vi "HFRR ADV v08 new software.vi"() -> ()   [LabVIEW 2025] (continued)
                  n3105 = Concatenate Strings(w4140, "=" ("string")) -> (→"String 37":string)
                }
                frame 43 {
                  n3106 = property on="HCF 2" class="DigNum (strict)"("Caption.Text"=w4143) -> ()  [unwired: 2 in, 2 out]
                  n3107 = property on="HCF" class="DigNum (strict)"("Caption.Text"=w4143) -> ()  [unwired: 2 in, 2 out]
                  n3108 = Concatenate Strings(w4143, "=" ("string")) -> (→"String 38":string)
                }
                frame 44 {
                  n3109 = Concatenate Strings(w4145, "=" ("string")) -> (→"String 39":string)
                  n3110 = property on="WS1.4 2" class="DigNum (strict)"("Caption.Text"=w4145) -> ()  [unwired: 2 in, 2 out]
                  n3111 = property on="WS1.4" class="DigNum (strict)"("Caption.Text"=w4145) -> ()  [unwired: 2 in, 2 out]
                }
                frame 45 {
                  n3112 = property on="Save Results" class="Bool (strict)"("Boolean Text.Text"=w4147) -> ()  [unwired: 2 in, 2 out]
                }
                frame 46 {
                  n3113 = local write "S 47"(w4148) -> ()
                }
                frame 47 {
                  n3114 = local write "S 48"(w4149) -> ()
                }
                frame 48 {
                  n3115 = local write "S 49"(w4150) -> ()
                }
                frame 49 {
                  n3116 = local write "S 50"(w4151) -> ()
                }
                frame 50 {
                  n3117 = local write "S 51"(w4152) -> ()
                }
                frame 51 {
                  n3118 = local write "S 52"(w4153) -> ()
                }
                frame 52 {
                  n3119 = local write "S 53"(w4154) -> ()
                }
                frame 53 {
                  n3120 = local write "S 54"(w4155) -> ()
                }
                frame 54 {
                  n3121 = local write "S 55"(w4156) -> ()
                }
                frame 55 {
                  n3122 = local write "S 56"(w4157) -> ()
                }
                frame 56 {
                  n3123 = local write "S 57"(w4158) -> ()
                }
                frame 57 {
                  n3124 = local write "S 58"(w4159) -> ()
                }
                frame 58 {
                  n3125 = local write "S 59"(w4160) -> ()
                }
                frame 59 {
                  n3126 = local write "S 60"(w4161) -> ()
                }
                frame 60 {
                  n3127 = local write "S 62"(w4162) -> ()
                }
                frame 61 {
                  n3128 = local write "S 63"(w4163) -> ()
                }
                frame 62 {
                  n3129 = local write "S 64"(w4164) -> ()
                }
                frame 63 {
                  n3130 = local write "S 65"(w4165) -> ()
                }
                frame 64 {
                  n3131 = local write "S 66"(w4166) -> ()
                }
                frame 65 {
                  n3132 = local write "S 67"(w4167) -> ()
                }
                frame 66 {
                  n3133 = local write "S 68"(w4168) -> ()
                }
                frame 67 {
                  n3134 = local write "S 69"(w4169) -> ()
                }
                frame 68 {
                  n3135 = local write "S 70"(w4170) -> ()
                }
                frame 69 {
                  n3136 = local write "S 71"(w4171) -> ()
                }
                frame 70 {
                  n3137 = local write "S 72"(w4172) -> ()
                }
                frame 71 {
                  n3138 = local write "S 73"(w4173) -> ()
                }
                frame 72 {
                  n3139 = local write "S 74"(w4174) -> ()
                }
                frame 73 {
                  n3140 = local write "S 75"(w4175) -> ()
                }
                frame 74 {
                  n3141 = local write "S 76"(w4176) -> ()
                }
                frame 75 {
                  n3142 = local write "S 77"(w4177) -> ()
                }
                frame 76 {
                  n3143 = local write "S 78"(w4178) -> ()
                }
                frame 77 {
                  n3144 = local write "S 79"(w4179) -> ()
                }
                frame 79 {
                  n3145 = property on="Sample Temperature ( °C )" class="XYGraph (strict)"("Y Scale.Name Label.Text"=w4180) -> ()  [unwired: 2 in, 2 out]
                }
                frame 80 {
                  n3146 = local write "S 81"(w4181) -> ()
                  n3147 = property on="Humidity ( %RH )" class="XYGraph (strict)"("Y Scale.Name Label.Text"=w4181) -> ()  [unwired: 2 in, 2 out]
                }
                frame 78 {
                  n3148 = property on="Air Temperature  ( °C )" class="XYGraph (strict)"("X Scale.Name Label.Text"=w4182) -> ()  [unwired: 2 in, 2 out]
                  n3149 = property on="Humidity ( %RH )" class="XYGraph (strict)"("X Scale.Name Label.Text"=w4182) -> ()  [unwired: 2 in, 2 out]
                  n3150 = property on="Sample Temperature ( °C )" class="XYGraph (strict)"("X Scale.Name Label.Text"=w4182) -> ()  [unwired: 2 in, 2 out]
                  n3151 = property on="Coefficient Of Friction" class="XYGraph (strict)"("X Scale.Name Label.Text"=w4182) -> ()  [unwired: 2 in, 2 out]
                }
                frame 81 {
                  n3152 = property on="Air Temperature  ( °C )" class="XYGraph (strict)"("Y Scale.Name Label.Text"=w4183) -> ()  [unwired: 2 in, 2 out]
                }
                frame 82 {
                  n3153 = local write "S 84"(w4184) -> ()
                }
                frame 83 {
                  n3154 = local write "S 85"(w4185) -> ()
                }
                frame 84 {
                  n3155 = local write "S 86"(w4186) -> ()
                }
                frame 85 {
                  n3156 = local write "S 87"(w4187) -> ()
                }
                frame 86 {
                  n3157 = local write "S 88"(w4188) -> ()
                }
                frame 87 {
                }
                frame 88 {
                  n3158 = local write "S 90"(w4190) -> ()
                }
                frame 89 {
                  n3159 = local write "S 91"(w4191) -> ()
                }
                frame 90 {
                  n3160 = local write "S 92"(w4192) -> ()
                }
                frame 91 {
                  n3161 = local write "S 93"(w4193) -> ()
                }
                frame 92 {
                  n3162 = local write "S 94"(w4194) -> ()
                }
                frame 93 {
                  n3163 = local write "S 95"(w4195) -> ()
                }
                frame 94 {
                  n3164 = local write "S 96"(w4196) -> ()
                }
                frame 95 {
                  n3165 = local write "S 97"(w4197) -> ()
                }
                frame 96 {
                  n3166 = local write "S 98"(w4198) -> ()
                }
                frame 97 {
                  n3167 = local write "S 99"(w4199) -> ()
                }
                frame 98 {
                  n3168 = local write "S 100"(w4200) -> ()
                }
                frame 99 {
                  n3169 = local write "S 101"(w4201) -> ()
                }
                frame 100 {
                  n3170 = local write "S 102"(w4202) -> ()
                }
                frame 101 {
                  n3171 = local write "S 103"(w4203) -> ()
                }
                frame 102 {
                  n3172 = local write "S 104"(w4204) -> ()
                }
                frame 103 {
                  n3173 = local write "S 105"(w4205) -> ()
                }
                frame 104 {
                  n3174 = local write "S 106"(w4206) -> ()
                }
                frame 105 {
                }
                frame 106 {
                  n3175 = property on="OK Button 17" class="Bool (strict)"("Boolean Text.Text"=w4207) -> ()  [unwired: 2 in, 2 out]
                }
                frame 107 {
                  n3176 = property on="OK Button 16" class="Bool (strict)"("Boolean Text.Text"=w4208) -> ()  [unwired: 2 in, 2 out]
                }
                frame 108 {
                  n3177 = property on="TITTLE" class="Str"("Caption.Text"=w4209) -> ()  [unwired: 2 in, 2 out]
                }
                frame 109 {
                  "String 30" <- w4210
                }
                frame 110 {
                  n3178 = property on="Test Date" class="Str"("Caption.Text"=w4211) -> ()  [unwired: 2 in, 2 out]
                  "String 31" <- w4211
                }
                frame 111 {
                  n3179 = property on="Sample ID" class="Str"("Caption.Text"=w4212) -> ()  [unwired: 2 in, 2 out]
                  "String 32" <- w4212
                }
                frame 112 {
                  n3180 = property on="Tested by" class="Str"("Caption.Text"=w4213) -> ()  [unwired: 2 in, 2 out]
                  "String 33" <- w4213
                }
                frame 113 {
                  n3181 = property on="System Configured Printers 2" class="Arr (strict)"("Caption.Text"=w4214) -> ()  [unwired: 2 in, 2 out]
                }
                frame 114 {
                  n3182 = property on="Selected Printer" class="Str"("Caption.Text"=w4215) -> ()  [unwired: 2 in, 2 out]
                }
                frame 115 {
                  n3183 = property on="Select Printer 3" class="DigNum (strict)"("Caption.Text"=w4216) -> ()  [unwired: 2 in, 2 out]
                }
                frame 116 {
                  n3184 = property on="Print" class="Bool (strict)"("Boolean Text.Text"=w4217) -> ()  [unwired: 2 in, 2 out]
                }
                frame 117 {
                  "String 41" <- w4218
                }
                frame 118 {
                  n3185 = property on="tested by" class="Str"("Caption.Text"=w4219) -> ()  [unwired: 2 in, 2 out]
                }
                frame 119 {
                }
                frame 120 {
                  n3186 = property on="Export" class="Bool (strict)"("Boolean Text.Text"=w4220) -> ()  [unwired: 2 in, 2 out]
                }
                frame 121 {
                  n3187 = property on="TEMP INTERCEPT:" class="DigNum (strict)"("Caption.Text"=w4221) -> ()  [unwired: 2 in, 2 out]
                }
                frame 122 {
                  n3188 = property on="AIR TEMP INTERCEPT:" class="DigNum (strict)"("Caption.Text"=w4222) -> ()  [unwired: 2 in, 2 out]
                }
                frame 123 {
                  n3189 = property on="Select File Type" class="Enum (strict)"("Caption.Text"=w4223) -> ()  [unwired: 2 in, 2 out]
                }
                frame 124 {
                  n3190 = property on="s.NO" class="Str"("Caption.Text"=w4224) -> ()  [unwired: 2 in, 2 out]
                  "String 45" <- w4224
                }
                frame 125 {
                  n3191 = property on="trip1 8" class="Bool (strict)"("Boolean Text.Text"=w4225) -> ()  [unwired: 2 in, 2 out]
                }
                frame 126, Default {
                }
              }
            }
          }
          frame #1 {
            w4233 = TRUE ("Visible")
            n3192 = local read "S 91"() -> (w4250:string)
            n3193 = local read "S 90"() -> (w4249:string)
            n3194 = local read "S 88"() -> (w4248:string)
            n3195 = property on="File Path" class="Path"("Caption.Text"=w4249) -> ()  [unwired: 2 in, 2 out]
            n3196 = property on="SrvM CP" class="Bool (strict)"("Boolean Text.Text"=w4248) -> ()  [unwired: 2 in, 2 out]
            n3197 = local read "S 71"() -> (w4243:string)
            n3198 = local read "S 86"() -> (w4245:string)
            n3199 = local read "S 85"() -> (w4246:string)
            n3200 = local read "S 87"() -> (w4244:string)
            n3201 = local read "S 84"() -> (w4247:string)
            n3202 = local read "S 103"() -> (w4232:string)
            n3203 = local read "S 104"() -> (w4231:string)
            n3204 = property on="ENTER THE NEW PASSWORD" class="Str"("Caption.Text"=w4244) -> ()  [unwired: 2 in, 2 out]
            n3205 = property on="Password" class="Str"("Caption.Text"=w4246) -> ()  [unwired: 2 in, 2 out]
            n3206 = property on="ENTER CURRENT PASSWORD" class="Str"("Caption.Text"=w4245) -> ()  [unwired: 2 in, 2 out]
            n3207 = property on="EDIT" class="Bool (strict)"("Boolean Text.Text"=w4243) -> ()  [unwired: 2 in, 2 out]
            n3208 = property on="SAVE" class="Bool (strict)"("Boolean Text.Text"=w4247) -> ()  [unwired: 2 in, 2 out]
            n3209 = Build Array(w4232, w4231) -> (w4230:string[])
            n3210 = property on="Heater Button" class="Bool (strict)"("Strings [4]"=w4230) -> ()  [unwired: 2 in, 2 out]
            n3211 = property on="CH-HUMIDITY WET" class="DigNum (strict)"("Caption.Size to Text?"=w4233) -> ()  [unwired: 2 in, 2 out]
            n3212 = property on="CH-HUMIDITY DRY" class="DigNum (strict)"("Caption.Size to Text?"=w4233) -> ()  [unwired: 2 in, 2 out]
            n3213 = property on="CH-POWER -" class="DigNum (strict)"("Caption.Size to Text?"=w4233) -> ()  [unwired: 2 in, 2 out]
            n3214 = property on="CH-HEATER" class="DigNum (strict)"("Caption.Size to Text?"=w4233) -> ()  [unwired: 2 in, 2 out]
            n3215 = property on="CH-POWER +" class="DigNum (strict)"("Caption.Size to Text?"=w4233) -> ()  [unwired: 2 in, 2 out]
            n3216 = local read "S 92"() -> (w4242:string)
            n3217 = local read "S 93"() -> (w4241:string)
            n3218 = local read "S 105"() -> (w4228:string)
            n3219 = local read "S 106"() -> (w4227:string)
            n3220 = Build Array(w4242, w4241) -> ()  [unwired: 1 out]
            n3221 = Build Array(w4228, w4227) -> (w4229:string[])
            n3222 = local read "S 95"() -> (w4239:string)
            n3223 = local read "S 94"() -> (w4240:string)
            n3224 = local read "bs"() -> (w4255:string)
            n3225 = local read "as"() -> (w4256:string)
            n3226 = property on="Humidity" class="Bool (strict)"("Strings [4]"=w4229) -> ()  [unwired: 2 in, 2 out]
            n3227 = Concatenate Strings(w4255, "\r", w4256) -> ()  [unwired: 1 out]
            n3228 = property on="STROKE GAIN :" class="DigNum (strict)"("Caption.Text"=w4239) -> ()  [unwired: 2 in, 2 out]
            n3229 = property on="DISPLACEMENT :" class="DigNum (strict)"("Caption.Text"=w4240) -> ()  [unwired: 2 in, 2 out]
            n3230 = property on="Rh After" class="DigNum (strict)"("Caption.Size to Text?"=TRUE ("Caption.Size to Text")) -> ()  [unwired: 2 in, 2 out]
            n3231 = local read "S 48"() -> (w4279:string)
            n3232 = local read "S 50"() -> (w4277:string)
            n3233 = local read "S 51"() -> (w4276:string)
            n3234 = local read "S 49"() -> (w4278:string)
            n3235 = local read "S 52"() -> (w4275:string)
            n3236 = local read "as"() -> (w4260:string)
            n3237 = local read "bs"() -> (w4261:string)
            n3238 = local read "S 56"() -> (w4274:string)
            n3239 = local read "S 57"() -> (w4273:string)
            n3240 = local read "S 58"() -> (w4272:string)
            n3241 = local read "S 59"() -> (w4271:string)
            n3242 = property on="OPEN" class="Bool (strict)"("Boolean Text.Text"=w4275) -> ()  [unwired: 2 in, 2 out]
            n3243 = property on="OPEN 1" class="Bool (strict)"("Boolean Text.Text"=w4279) -> ()  [unwired: 2 in, 2 out]
            n3244 = property on="OPEN 2" class="Bool (strict)"("Boolean Text.Text"=w4278) -> ()  [unwired: 2 in, 2 out]
            n3245 = property on="OPEN 3" class="Bool (strict)"("Boolean Text.Text"=w4277) -> ()  [unwired: 2 in, 2 out]
            n3246 = property on="OPEN 4" class="Bool (strict)"("Boolean Text.Text"=w4276) -> ()  [unwired: 2 in, 2 out]
            n3247 = Concatenate Strings(w4261, "\r", w4260) -> ()  [unwired: 1 out]
            n3248 = local read "S 102"() -> (w4234:string)
            n3249 = property on="КОФ1" class="DigNum (strict)"("Caption.Text"=w4274) -> ()  [unwired: 2 in, 2 out]
            n3250 = local read "S 98"() -> (w4238:string)
            n3251 = local read "S 99"() -> (w4237:string)
            n3252 = local read "S 100"() -> (w4236:string)
            n3253 = local read "S 101"() -> (w4235:string)
            n3254 = property on="КОФ2" class="DigNum (strict)"("Caption.Text"=w4273) -> ()  [unwired: 2 in, 2 out]
            n3255 = property on="КОФ3" class="DigNum (strict)"("Caption.Text"=w4272) -> ()  [unwired: 2 in, 2 out]
            n3256 = property on="КОФ4" class="DigNum (strict)"("Caption.Text"=w4271) -> ()  [unwired: 2 in, 2 out]
            n3257 = local read "bs"() -> (w4259:string)
            n3258 = local read "as"() -> (w4258:string)
            n3259 = property on="CH-POWER +" class="DigNum (strict)"("Caption.Text"=w4238) -> ()  [unwired: 2 in, 2 out]
            n3260 = property on="CH-POWER -" class="DigNum (strict)"("Caption.Text"=w4237) -> ()  [unwired: 2 in, 2 out]
            n3261 = property on="CH-HEATER" class="DigNum (strict)"("Caption.Text"=w4236) -> ()  [unwired: 2 in, 2 out]
            n3262 = property on="CH-HUMIDITY DRY" class="DigNum (strict)"("Caption.Text"=w4235) -> ()  [unwired: 2 in, 2 out]
            n3263 = property on="CH-HUMIDITY WET" class="DigNum (strict)"("Caption.Text"=w4234) -> ()  [unwired: 2 in, 2 out]
            n3264 = local read "S 60"() -> (w4270:string)
            n3265 = local read "S 54"() -> (w4280:string)
            n3266 = Concatenate Strings(w4259, "\r", w4258) -> ()  [unwired: 1 out]
            n3267 = Concatenate Strings(w4280, w4270) -> ()  [unwired: 1 out]
            n3268 = local read "S 77"() -> (→"String 43":string)
            n3269 = local read "S 76"() -> (w4253:string)
            n3270 = local read "S 78"() -> (w4252:string)
            n3271 = local read "S 71"() -> (w4264:string)
            n3272 = local read "S 66"() -> (w4269:string)
            n3273 = local read "S 67"() -> (w4268:string)
            n3274 = local read "S 68"() -> (w4267:string)
            n3275 = local read "S 69"() -> (w4266:string)
            n3276 = local read "S 70"() -> (w4265:string)
            n3277 = property on="AIR TEMP" class="DigNum (strict)"("Caption.Text"=w4252) -> ()  [unwired: 2 in, 2 out]
            n3278 = property on="Set Strk" class="DigNum (strict)"("Caption.Text"=w4253) -> ()  [unwired: 2 in, 2 out]
            n3279 = property on="FRIC. FORCE :" class="DigNum (strict)"("Caption.Text"=w4269) -> ()  [unwired: 2 in, 2 out]
            n3280 = property on="TEMPERATURE :" class="DigNum (strict)"("Caption.Text"=w4268) -> ()  [unwired: 2 in, 2 out]
            n3281 = property on="SPEED OUT:" class="DigNum (strict)"("Caption.Text"=w4267) -> ()  [unwired: 2 in, 2 out]
            n3282 = property on="AIR TEMPERATURE :" class="DigNum (strict)"("Caption.Text"=w4266) -> ()  [unwired: 2 in, 2 out]
            n3283 = property on="HUMIDITY:" class="DigNum (strict)"("Caption.Text"=w4265) -> ()  [unwired: 2 in, 2 out]
            n3284 = property on="EDIT" class="Bool (strict)"("Boolean Text.Text"=w4264) -> ()  [unwired: 2 in, 2 out]
            n3285 = local read "S 79"() -> (w4251:string)
          }
          frame #2 {
          }
        }
        n3286 = local write "Lan flag"(10.0 ("Lan flag")) -> ()
      }
      frame Enabled {
      }
    }
    n3287 = Wait (ms)(milliseconds to wait=u32 2000) -> ()  [unwired: 1 out]
    n3288 = local read "Quit"() -> (w4054:bool)
  }
  n3289 = disable-structure shown="Disabled" {
    frame Disabled {
      n3290 = while {
        tunnel: [w4282] -> _
        i -> [w4282]
        stop <- w4281 continue-if-true
        n3291 = Wait (ms)(milliseconds to wait=u32 50) -> ()  [unwired: 1 out]
        n3292 = stacked-sequence {
          frame #0 {
            # "Controls Text color"
            # "Controls BG color"
            n3293 = property on="FILE" class="Str"("Text.Text Colors:Text Color"="SC  Text") -> ()  [unwired: 2 in, 2 out]
            n3294 = property on="Fuel Discription :" class="Str"("Text.Text Colors:Text Color"="SC  Text") -> ()  [unwired: 2 in, 2 out]
            n3295 = property on="tested by" class="Str"("Text.Text Colors:Text Color"="SC  Text") -> ()  [unwired: 2 in, 2 out]
            n3296 = property on="Remarks :" class="Str"("Text.Text Colors:Text Color"="SC  Text") -> ()  [unwired: 2 in, 2 out]
            n3297 = property class="DigNum (strict)"("Numeric Text.Text Colors:BG Color"="NC BG") -> ()  [unwired: 2 in, 2 out]
            n3298 = property class="DigNum (strict)"("Numeric Text.Text Colors:BG Color"="NC BG") -> ()  [unwired: 2 in, 2 out]
            n3299 = property class="DigNum (strict)"("Numeric Text.Text Colors:BG Color"="NC BG") -> ()  [unwired: 2 in, 2 out]
            n3300 = property class="DigNum (strict)"("Numeric Text.Text Colors:BG Color"="NC BG") -> ()  [unwired: 2 in, 2 out]
            n3301 = property class="DigNum (strict)"("Numeric Text.Text Colors:BG Color"="NC BG") -> ()  [unwired: 2 in, 2 out]
            n3302 = property class="DigNum (strict)"("Numeric Text.Text Colors:BG Color"="NC BG") -> ()  [unwired: 2 in, 2 out]
            n3303 = property class="DigNum (strict)"("Numeric Text.Text Colors:BG Color"="NC BG") -> ()  [unwired: 2 in, 2 out]
            n3304 = property class="DigNum (strict)"("Numeric Text.Text Colors:BG Color"="NC BG") -> ()  [unwired: 2 in, 2 out]
            n3305 = property class="DigNum (strict)"("Numeric Text.Text Colors:BG Color"="NC BG") -> ()  [unwired: 2 in, 2 out]
            n3306 = property class="DigNum (strict)"("Numeric Text.Text Colors:BG Color"="NC BG") -> ()  [unwired: 2 in, 2 out]
            n3307 = property class="DigNum (strict)"("Numeric Text.Text Colors:BG Color"="NC BG") -> ()  [unwired: 2 in, 2 out]
            n3308 = property class="DigNum (strict)"("Numeric Text.Text Colors:BG Color"="NC BG") -> ()  [unwired: 2 in, 2 out]
            n3309 = property on="FILE" class="Str"("Text.Text Colors:BG Color"="SC BG 3") -> ()  [unwired: 2 in, 2 out]
            n3310 = property on="Fuel Discription :" class="Str"("Text.Text Colors:BG Color"="SC BG 3") -> ()  [unwired: 2 in, 2 out]
            n3311 = property on="tested by" class="Str"("Text.Text Colors:BG Color"="SC BG 3") -> ()  [unwired: 2 in, 2 out]
            n3312 = property on="Remarks :" class="Str"("Text.Text Colors:BG Color"="SC BG 3") -> ()  [unwired: 2 in, 2 out]
            n3313 = property class="DigNum (strict)"("Numeric Text.Text Colors:Text Color"="NC Text") -> ()  [unwired: 2 in, 2 out]
            n3314 = property class="DigNum (strict)"("Numeric Text.Text Colors:Text Color"="NC Text") -> ()  [unwired: 2 in, 2 out]
            n3315 = property class="DigNum (strict)"("Numeric Text.Text Colors:Text Color"="NC Text") -> ()  [unwired: 2 in, 2 out]
            n3316 = property class="DigNum (strict)"("Numeric Text.Text Colors:Text Color"="NC Text") -> ()  [unwired: 2 in, 2 out]
            n3317 = property class="DigNum (strict)"("Numeric Text.Text Colors:Text Color"="NC Text") -> ()  [unwired: 2 in, 2 out]
            n3318 = property class="DigNum (strict)"("Numeric Text.Text Colors:Text Color"="NC Text") -> ()  [unwired: 2 in, 2 out]
            n3319 = property class="DigNum (strict)"("Numeric Text.Text Colors:Text Color"="NC Text") -> ()  [unwired: 2 in, 2 out]
            n3320 = property class="DigNum (strict)"("Numeric Text.Text Colors:Text Color"="NC Text") -> ()  [unwired: 2 in, 2 out]
            n3321 = property class="DigNum (strict)"("Numeric Text.Text Colors:Text Color"="NC Text") -> ()  [unwired: 2 in, 2 out]
            n3322 = property class="DigNum (strict)"("Numeric Text.Text Colors:Text Color"="NC Text") -> ()  [unwired: 2 in, 2 out]
            n3323 = property class="DigNum (strict)"("Numeric Text.Text Colors:Text Color"="NC Text") -> ()  [unwired: 2 in, 2 out]
            n3324 = property class="DigNum (strict)"("Numeric Text.Text Colors:Text Color"="NC Text") -> ()  [unwired: 2 in, 2 out]
            n3325 = property class="DigNum (strict)"("Numeric Text.Text Colors:Text Color"="NI Text  2") -> ()  [unwired: 2 in, 2 out]
            n3326 = property class="DigNum (strict)"("Numeric Text.Text Colors:Text Color"="NI Text  2") -> ()  [unwired: 2 in, 2 out]
            n3327 = property class="DigNum (strict)"("Numeric Text.Text Colors:Text Color"="NI Text  2") -> ()  [unwired: 2 in, 2 out]
            n3328 = property class="DigNum (strict)"("Numeric Text.Text Colors:Text Color"="NI Text  2") -> ()  [unwired: 2 in, 2 out]
            n3329 = property class="DigNum (strict)"("Numeric Text.Text Colors:Text Color"="NI Text  2") -> ()  [unwired: 2 in, 2 out]
            n3330 = property class="DigNum (strict)"("Numeric Text.Text Colors:Text Color"="NI Text  2") -> ()  [unwired: 2 in, 2 out]
            n3331 = property class="DigNum (strict)"("Numeric Text.Text Colors:Text Color"="NI Text  2") -> ()  [unwired: 2 in, 2 out]
            n3332 = property class="DigNum (strict)"("Numeric Text.Text Colors:Text Color"="NI Text  2") -> ()  [unwired: 2 in, 2 out]
            n3333 = property class="DigNum (strict)"("Numeric Text.Text Colors:Text Color"="NI Text  2") -> ()  [unwired: 2 in, 2 out]
            n3334 = property class="DigNum (strict)"("Numeric Text.Text Colors:Text Color"="NI Text  2") -> ()  [unwired: 2 in, 2 out]
            n3335 = property class="DigNum (strict)"("Numeric Text.Text Colors:Text Color"="NI Text  2") -> ()  [unwired: 2 in, 2 out]
            n3336 = property class="DigNum (strict)"("Numeric Text.Text Colors:Text Color"="NI Text  2") -> ()  [unwired: 2 in, 2 out]
            n3337 = property class="DigNum (strict)"("Numeric Text.Text Colors:Text Color"="NI Text  2") -> ()  [unwired: 2 in, 2 out]
            n3338 = property class="DigNum (strict)"("Numeric Text.Text Colors:Text Color"="NI Text  2") -> ()  [unwired: 2 in, 2 out]
            n3339 = property class="DigNum (strict)"("Numeric Text.Text Colors:Text Color"="NI Text  2") -> ()  [unwired: 2 in, 2 out]
            n3340 = property on="Coefficient Of Friction" class="XYGraph (strict)"("Plot Area:Colors:FG Color"="GFG  2", "Plot Area:Colors:BG Color"="GBG   2") -> ()  [unwired: 2 in, 2 out]
            n3341 = property on="Humidity ( %RH )" class="XYGraph (strict)"("Plot Area:Colors:FG Color"="GFG  2", "Plot Area:Colors:BG Color"="GBG   2") -> ()  [unwired: 2 in, 2 out]
            n3342 = property on="Air Temperature  ( °C )" class="XYGraph (strict)"("Plot Area:Colors:FG Color"="GFG  2", "Plot Area:Colors:BG Color"="GBG   2") -> ()  [unwired: 2 in, 2 out]
            n3343 = property on="Sample Temperature ( °C )" class="XYGraph (strict)"("Plot Area:Colors:FG Color"="GFG  2", "Plot Area:Colors:BG Color"="GBG   2") -> ()  [unwired: 2 in, 2 out]
            n3344 = property class="DigNum (strict)"("Numeric Text.Text Colors:BG Color"="NI BG 2") -> ()  [unwired: 2 in, 2 out]
            n3345 = property class="DigNum (strict)"("Numeric Text.Text Colors:BG Color"="NI BG 2") -> ()  [unwired: 2 in, 2 out]
            n3346 = property class="DigNum (strict)"("Numeric Text.Text Colors:BG Color"="NI BG 2") -> ()  [unwired: 2 in, 2 out]
            n3347 = property class="DigNum (strict)"("Numeric Text.Text Colors:BG Color"="NI BG 2") -> ()  [unwired: 2 in, 2 out]
            n3348 = property class="DigNum (strict)"("Numeric Text.Text Colors:BG Color"="NI BG 2") -> ()  [unwired: 2 in, 2 out]
            n3349 = property class="DigNum (strict)"("Numeric Text.Text Colors:BG Color"="NI BG 2") -> ()  [unwired: 2 in, 2 out]
            n3350 = property class="DigNum (strict)"("Numeric Text.Text Colors:BG Color"="NI BG 2") -> ()  [unwired: 2 in, 2 out]
            n3351 = property class="DigNum (strict)"("Numeric Text.Text Colors:BG Color"="NI BG 2") -> ()  [unwired: 2 in, 2 out]
            n3352 = property class="DigNum (strict)"("Numeric Text.Text Colors:BG Color"="NI BG 2") -> ()  [unwired: 2 in, 2 out]
            n3353 = property class="DigNum (strict)"("Numeric Text.Text Colors:BG Color"="NI BG 2") -> ()  [unwired: 2 in, 2 out]
            n3354 = property class="DigNum (strict)"("Numeric Text.Text Colors:BG Color"="NI BG 2") -> ()  [unwired: 2 in, 2 out]
            n3355 = property class="DigNum (strict)"("Numeric Text.Text Colors:BG Color"="NI BG 2") -> ()  [unwired: 2 in, 2 out]
            n3356 = property class="DigNum (strict)"("Numeric Text.Text Colors:BG Color"="NI BG 2") -> ()  [unwired: 2 in, 2 out]
            n3357 = property class="DigNum (strict)"("Numeric Text.Text Colors:BG Color"="NI BG 2") -> ()  [unwired: 2 in, 2 out]
            n3358 = property class="DigNum (strict)"("Numeric Text.Text Colors:BG Color"="NI BG 2") -> ()  [unwired: 2 in, 2 out]
            n3359 = property class="Bool"("Colors [4]"="Boolean BC T & BG") -> ()  [unwired: 2 in, 2 out]
            n3360 = property on="Save & Continue" class="Bool (strict)"("Colors [4]"="Boolean BC T & BG") -> ()  [unwired: 2 in, 2 out]
            n3361 = property on="Heater Button" class="Bool (strict)"("Colors [4]"="Boolean BC T & BG") -> ()  [unwired: 2 in, 2 out]
            n3362 = property class="Bool"("Colors [4]"="Boolean BC T & BG") -> ()  [unwired: 2 in, 2 out]
            n3363 = property on="Humidity" class="Bool (strict)"("Colors [4]"="Boolean BC T & BG") -> ()  [unwired: 2 in, 2 out]
            n3364 = property class="Bool (strict)"("Colors [4]"="Boolean BC T & BG") -> ()  [unwired: 2 in, 2 out]
            n3365 = property on="RUN" class="Bool (strict)"("Colors [4]"="Boolean BC T & BG") -> ()  [unwired: 2 in, 2 out]
            n3366 = property on="trip1 8" class="Bool (strict)"("Colors [4]"="Boolean BC T & BG") -> ()  [unwired: 2 in, 2 out]
            n3367 = property class="Bool"("Colors [4]"="Boolean BC T & BG") -> ()  [unwired: 2 in, 2 out]
            n3368 = property class="Bool (strict)"("Colors [4]"="Boolean BC T & BG") -> ()  [unwired: 2 in, 2 out]
            n3369 = property on="OPEN 1" class="Bool (strict)"("Colors [4]"="Boolean BC T & BG 2") -> ()  [unwired: 2 in, 2 out]
            n3370 = property on="OPEN 2" class="Bool (strict)"("Colors [4]"="Boolean BC T & BG 2") -> ()  [unwired: 2 in, 2 out]
            n3371 = property on="OPEN 3" class="Bool (strict)"("Colors [4]"="Boolean BC T & BG 2") -> ()  [unwired: 2 in, 2 out]
            n3372 = property on="OPEN 4" class="Bool (strict)"("Colors [4]"="Boolean BC T & BG 2") -> ()  [unwired: 2 in, 2 out]
            n3373 = property on="OPEN" class="Bool (strict)"("Colors [4]"="Boolean BC T & BG 2") -> ()  [unwired: 2 in, 2 out]
            n3374 = property on="rstv2" class="Bool"("Colors [4]"="Boolean BC T & BG 2") -> ()  [unwired: 2 in, 2 out]
            n3375 = property on="RST CP" class="Bool"("Colors [4]"="Boolean BC T & BG 2") -> ()  [unwired: 2 in, 2 out]
            n3376 = property on="RSTV1 3" class="Bool"("Colors [4]"="Boolean BC T & BG 2") -> ()  [unwired: 2 in, 2 out]
            n3377 = property on="RSTV1 2" class="Bool"("Colors [4]"="Boolean BC T & BG 2") -> ()  [unwired: 2 in, 2 out]
          }
          frame #1 {
          }
        }
        n3378 = local read "Quit"() -> (w4281:bool)
      }
    }
    frame Enabled {
    }
  }
  n3379 = while {
    shift-right: [w4299] -> _
    shift-left: _ -> [w4300]
    shift-right: [w4297] -> _
    shift-left: T17 {"Read Heave and Surge"="", "Bytes at Heave Port"=0.0, "Heave and Surge COM Port:"="COM9", "Com Port 2"="COM7", "Residual Due"="", "Heave COM Status 2"=TRUE, "Heave COM Status"=TRUE, "Port 2"=TRUE, "Sway PPR"=6400.0, "Surge PPR"=6400.0, "Heave PPR"=6400.0, "Sway Pitch"=2.0, "Surge Pitch"=3.0, "Heave Pitch"=4.0, "Sway Pulses/mm"=320.0, "Surge Pulses/mm"=1600.0, "Heave Pulses/mm"=1600.0, "inner loop"=0.0, "Read Heave and Surge 2"="", "String 36"="", "Write S"=FALSE, "WriteCC1"=[""], "Heave COM Loop"=0, "LastCom"="", "EXIT"=FALSE, "Error Heave"={"status"=TRUE, "code"=-1073807343, "source"=""}} -> [w4296]
    shift-right: [w4294] -> _
    shift-left: enum16{"init", "MAIN", "Panel Close"}."init" -> [w4295]
    stop <- w4298 stop-if-true
    n3380 = case shown="\"MAIN\"" w4295 {
      tunnel: w4300 -> [w4314 w4329 w4390 w4392]
      tunnel: [w4308 w4338 w4390 w4392] -> w4299
      tunnel: [_ _ TRUE _] -> w4298
      tunnel: [w4304 w4335 w4388 w4391] -> w4297
      tunnel: w4296 -> [w4311 w4328 w4388 w4391]
      tunnel: [enum16{"init", "MAIN", "Panel Close"}."MAIN" w4322 _ _] -> w4294
      frame "init" {
        n3381 = Bundle By Name(cluster=w4311, "Heave and Surge COM Port:"="C3 :") -> (w4310:T17)
        n3382 = call "Instrument fgv.vi"("Enum"=T29."INIT", "error in (no error) 2"=w4314, "INPUT"=w4310) -> ("error"=w4312:errorcluster, "output"=w4307:T17)  [unwired: 6 in, 1 out]
        n3383 = case shown="No Error" w4312 {
          selector: w4312 -> [w4316 _]
          tunnel: [w4316 w4320] -> w4308
          tunnel: w4307 -> [w4315 w4318]
          tunnel: [w4315 w4317] -> w4305
          frame No Error {
          }
          frame Error {
            n3384 = call "Instrument fgv.vi"("Enum"=T29."ERROR INIT", "INPUT"=w4318) -> ("error"=w4321:errorcluster, "output"=w4317:T17)  [unwired: 7 in, 1 out]
            n3385 = call <vilib>:"Clear Errors.vi"("error in (no error)"=w4321) -> ("error out"=w4320:errorcluster)  [unwired: 5 in, 1 out]
          }
        }
        n3386 = local read "LastCom"() -> (w4303:string)
        n3387 = Unbundle By Name(w4305) -> ("Heave COM Status 2"=→"COM Status" →"Instrument Status":bool, "Error Heave"=→"Error":errorcluster)  [unwired: 1 out]
        n3388 = Bundle By Name(cluster=w4305, "LastCom"=w4303) -> (w4304:T17)
      }
      frame "MAIN" {
        n3389 = Unbundle By Name(w4328) -> ("Com Port 2"=w4340:refnum<visa-resource-name>)
        n3390 = local write "Com Port 4"(w4340) -> ()
        n3391 = local read "C3 :"() -> (w4326:refnum<visa-resource-name>)
        n3392 = Bundle By Name(cluster=w4328, "Heave and Surge COM Port:"=w4326) -> (w4327:T17)
        n3393 = Equal?(x=w4340, y=w4326) -> (x = y?=w4339:bool)
        n3394 = case shown="True" w4339 {
          tunnel: [w4344 w4361] -> w4338
          tunnel: w4329 -> [w4345 w4367]
          tunnel: w4327 -> [w4343 w4365]
          tunnel: [w4342 w4360] -> w4335
          frame False {
            n3395 = call <vilib>:"Clear Errors.vi"("error in (no error)"=w4345) -> ("error out"=w4341:errorcluster)  [unwired: 5 in, 1 out]
            n3396 = call "Instrument fgv.vi"("Enum"=T29."ERROR INIT", "error in (no error) 2"=w4341, "INPUT"=w4343) -> ("error"=w4347:errorcluster, "output"=w4342:T17)  [unwired: 6 in, 1 out]
            n3397 = call <vilib>:"Clear Errors.vi"("error in (no error)"=w4347) -> ("error out"=w4344:errorcluster)  [unwired: 5 in, 1 out]
          }
          frame True {
            n3398 = call "Instrument fgv.vi"("Enum"=T29."READ", "error in (no error) 2"=w4367, "INPUT"=w4365) -> ("error"=w4366:errorcluster, "output"=w4357:T17)  [unwired: 6 in, 1 out]
            n3399 = Bundle By Name(cluster=w4357, "String 36"="String 11") -> (w4356:T17)
            n3400 = case shown="True" "Write S" {
              selector: "Write S" -> [_ w4387]
              tunnel: w4366 -> [w4380 w4386]
              tunnel: [w4380 w4385] -> w4353
              tunnel: w4356 -> [w4379 w4382]
              tunnel: [w4379 w4381] -> w4352
              frame False {
              }
              frame True {
                n3401 = Not(x=w4387) -> (.not. x?=w4383:bool)
                n3402 = local write "Write S"(w4383) -> ()
                n3403 = call "Instrument fgv.vi"("Enum"=T29."MANUAL WRITE", "error in (no error) 2"=w4386, "INPUT"=w4382) -> ("error"=w4385:errorcluster, "output"=w4381:T17)  [unwired: 6 in, 1 out]
              }
            }
            n3404 = Array Size(array="WriteHumidity") -> (size(s)=w4350:i32)
            n3405 = Greater Than 0?(x=w4350) -> (x > 0?=w4348:bool)
            n3406 = call "Instrument fgv.vi"("Enum"=T29."WRITE", "error in (no error) 2"=w4353, "WriteCC1"="WriteHumidity", "INPUT"=w4352) -> ("error"=w4363:errorcluster, "WriteCC1 2"=w4351:string[], "output"=w4362:T17)  [unwired: 5 in]
            n3407 = case shown="True" w4348 {
              tunnel: w4351 -> [_ w4369]
              frame False {
              }
              frame True {
                n3408 = local write "WriteHumidity"(w4369) -> ()
              }
            }
            n3409 = case shown="Error" w4363 {
              selector: w4363 -> [w4370 w4373]
              tunnel: w4362 -> [w4371 w4378]
              tunnel: [w4371 w4377] -> w4360
              tunnel: [w4370 w4375] -> w4361
              frame No Error {
              }
              frame Error {
                n3410 = call <vilib>:"Clear Errors.vi"("error in (no error)"=w4373) -> ("error out"=w4372:errorcluster)  [unwired: 5 in, 1 out]
                n3411 = call "Instrument fgv.vi"("Enum"=T29."ERROR INIT", "error in (no error) 2"=w4372, "INPUT"=w4378) -> ("error"=w4376:errorcluster, "output"=w4377:T17)  [unwired: 6 in, 1 out]
                n3412 = call <vilib>:"Clear Errors.vi"("error in (no error)"=w4376) -> ("error out"=w4375:errorcluster)  [unwired: 5 in, 1 out]
              }
            }
            n3413 = Unbundle By Name(w4360) -> ("LastCom"=→"LastCom":string, "Read Heave and Surge"=→"Read Humidity":string)
          }
        }
        n3414 = Unbundle By Name(w4335) -> ("Heave COM Status 2"=w4337:bool, "Heave COM Status"=w4336:bool, "Error Heave"=w4333:errorcluster, "Bytes at Heave Port"=→"Bytes at Humidity Port":dbl)
        n3415 = Unbundle By Name(w4333) -> ("status"=→"Humidity Port":bool)
        n3416 = Not(x=w4336) -> (.not. x?=w4330:bool)
        n3417 = local write "Error"(w4333) -> ()
        n3418 = Not(x=w4337) -> (.not. x?=w4331:bool)
        n3419 = local write "Instrument Status"(w4330) -> ()
        n3420 = local write "COM Status"(w4331) -> ()
        n3421 = local read "Quit"() -> (w4323:bool)
        n3422 = Select(t=enum16{"init", "MAIN", "Panel Close"}."Panel Close", s=w4323, f=enum16{"init", "MAIN", "Panel Close"}."MAIN") -> (s? t:f=w4322:enum16{"init", "MAIN", "Panel Close"})
      }
      frame "Panel Close" {
      }
      frame Default {
      }
    }
  }
  n3423 = while {
    stop <- w4418 stop-if-true
    n3424 = local read "Read Humidity"() -> (w4399:string)
    n3425 = call <vilib>:"High Resolution Polling Wait.vi"("seconds to wait"=0.1) -> ()  [unwired: 10 in, 1 out]
    n3426 = Spreadsheet String To Array(delimiter (Tab)=",", format string="", spreadsheet string=w4399, array type (2D Dbl)=string[] []) -> (array=w4413:string[])
    n3427 = for {
      tunnel: w4413 -> [w4423] mode=indexing
      tunnel: string[] ["STATE;", "SET;", "RH;", "T;", "AMB_RH;", "AMB_T;", "PUMP;", "FAN_IN;", "FAN_OUT;", "DEHUM;", "CURRENT;", "STALL;"] -> [w4422] mode=indexing
      tunnel: [w4421] -> w4412 mode=indexing
      n3428 = Match Pattern(string=w4423, regular expression=w4422) -> (after substring=w4421:string)  [unwired: 1 in, 3 out]
    }
    n3429 = Index Array(array=w4412) -> (element #1=→"STATE :":string, element #2=→"SET :":string, element #3=w4401:string, element #4=→"T :":string, element #5=w4398:string, element #6=→"AMB_T :":string, element #7=→"PUMP :":string, element #8=→"FAN_IN :":string, element #9=→"FAN_OUT :":string, element #10=→"DEHUM :":string, element #11=→"CURRENT :":string, element #12=→"STALL :":string)  [unwired: 12 in]
    "RH :" <- w4401
    "AMB_RH :" <- w4398
    n3430 = Fract/Exp String To Number(string=w4401) -> (number=w4393:dbl)  [unwired: 3 in, 1 out]
    n3431 = Fract/Exp String To Number(string=w4398) -> (number=w4397:dbl)  [unwired: 3 in, 1 out]
    n3432 = local write "Ambient Humidity :"(w4397) -> ()
    n3433 = Equal?(x=w4393, y=0.0) -> (x = y?=w4395:bool)
    n3434 = case shown="True" w4395 {
      tunnel: [w4419 w4420] -> w4394
      tunnel: w4393 -> [w4419 _]
      frame False {
        (unwired) 0.0
        "Humidity temp" <- w4419
      }
      frame True {
        n3435 = local read "Humidity temp"() -> (w4420:dbl)
      }
    }
    "RH Numeric:" <- w4394
    n3436 = local read "Quit"() -> (w4418:bool)
  }
  n3437 = disable-structure shown="Disabled" {
    frame Disabled {
      n3438 = while {
        tunnel: [w4657] -> _
        i -> [w4657]
        stop <- w4654 stop-if-true
        n3439 = local read "powstat"() -> (w4655:bool)
        n3440 = case shown="True" w4655 {
          frame False {
          }
          frame True {
            n3441 = local read "RUN"() -> (w4658:bool)
            n3442 = case shown="True" w4658 {
              frame False {
                w4688 = 65.0 ("y")
                n3443 = local read "Set Hz"() -> (w4716:dbl)
                n3444 = local read "NORMAL LOAD"() -> (w4717:dbl)
                n3445 = Multiply(x=w4716, y=60.0) -> (x*y=w4723:dbl)
                n3446 = Multiply(x=1.2 ("y"), y=0.949) -> (x*y=w4692:dbl)
                n3447 = Multiply(x=1.2 ("y"), y=0.8166) -> (x*y=w4696:dbl)
                n3448 = Multiply(x=1.2 ("y"), y=0.851) -> (x*y=w4691:dbl)
                n3449 = local read "FF 2"() -> (w4715:dbl)
                n3450 = Absolute Value(x=w4723) -> (abs(x)=w4721:dbl)
                n3451 = case shown="13.." w4715 {
                  tunnel: [1 2 3] -> w4713
                  frame 0..10, Default {
                    # "Normal"
                  }
                  frame 11, 12 {
                  }
                  frame 13.. {
                  }
                }
                "FF STATE" <- w4713
                n3452 = local read "TEMP"() -> (w4676:dbl)
                n3453 = local read item#-1() -> (w4690)
                n3454 = Less?(x=w4690, y=w4696) -> (x < y?=w4693:bool)
                n3455 = In Range and Coerce(upper limit=w4692, x=w4690, lower limit=w4691) -> (In Range?=w4694:bool)  [unwired: 1 out]
                n3456 = case shown="3601.." w4721 {
                  tunnel: [1 2 3] -> w4719
                  frame 0..3000, Default {
                    # "Normal"
                  }
                  frame 3001..3600 {
                  }
                  frame 3601.. {
                  }
                }
                n3457 = case shown="11.." w4717 {
                  tunnel: [1 3] -> w4718
                  frame 1..10, Default {
                  }
                  frame 11.. {
                  }
                }
                "NL STATE" <- w4718
                n3458 = Multiply(x=1.2 ("y"), y=0.95) -> (x*y=w4706:dbl)
                n3459 = Multiply(x=w4688, y=0.954) -> (x*y=w4680:dbl)
                n3460 = Or(x=w4693, y=w4694) -> (x .or. y?=w4695:bool)
                n3461 = Greater Or Equal?(x=w4690, y=w4706) -> (x >= y?=w4703:bool)
                n3462 = Multiply(x=w4688, y=0.99) -> (x*y=w4677:dbl)
                n3463 = Greater Or Equal?(x=w4676, y=w4677) -> (x >= y?=w4682:bool)
                n3464 = Greater Or Equal?(x=w4676, y=w4680) -> (x >= y?=w4679:bool)
                n3465 = case shown="0, 1, Default" w4690 {
                  tunnel: [1 3] -> w4707
                  frame 0, 1, Default {
                  }
                  frame 2.. {
                  }
                }
                n3466 = case shown="True" w4703 {
                  tunnel: [1 3] -> w4708
                  frame False {
                  }
                  frame True {
                  }
                }
                n3467 = case shown="True" w4695 {
                  tunnel: [1 2] -> w4709
                  frame False {
                  }
                  frame True {
                  }
                }
                n3468 = case shown="..0" w4676 {
                  tunnel: [2 3 3 1] -> w4683
                  frame 61, 62 {
                  }
                  frame 63.. {
                  }
                  frame ..0 {
                  }
                  frame 10..60, Default {
                  }
                }
                n3469 = case shown="True" w4682 {
                  tunnel: [1 3] -> w4684
                  frame False {
                  }
                  frame True {
                  }
                }
                n3470 = Number To Decimal String(number=w4719) -> (decimal integer string=w4720:string)  [unwired: 1 in]
                n3471 = case shown="True" w4679 {
                  tunnel: [1 2] -> w4685
                  frame False {
                  }
                  frame True {
                  }
                }
                n3472 = Number To Decimal String(number=1) -> (decimal integer string=→"Air temp":string)  [unwired: 1 in]
                n3473 = Number To Decimal String(number=w4713) -> (decimal integer string=→"ff_st":string)  [unwired: 1 in]
                n3474 = local write "sp_st"(w4720) -> ()
                n3475 = Number To Decimal String(number=w4718) -> (decimal integer string=→"nl_st":string)  [unwired: 1 in]
                n3476 = Build Array(w4683, w4684, w4685) -> (w4686:i32[])
                n3477 = Build Array(w4707, w4708, w4709) -> (w4710:i32[])
                n3478 = Array Max & Min(array=w4686) -> (max value=w4687:i32)  [unwired: 3 out]
                n3479 = Array Max & Min(array=w4710) -> (max value=w4711:i32)  [unwired: 3 out]
                n3480 = Number To Decimal String(number=w4687) -> (decimal integer string=w4675:string)  [unwired: 1 in]
                n3481 = Number To Decimal String(number=w4711) -> (decimal integer string=→"Stroke Ln 2":string)  [unwired: 1 in]
                n3482 = local write "temp_st"(w4675) -> ()
              }
              frame True {
                w4773 = 65.0 ("y")
                # "Healthy -1\nWarning -2\nError -3"
                n3483 = local read "TEMP"() -> (w4784:dbl)
                n3484 = local read "NORMAL LOAD"() -> (w4788:dbl)
                n3485 = local read "Set Hz"() -> (w4786:dbl)
                n3486 = Multiply(x=1.2 ("y"), y=0.949) -> (x*y=w4768:dbl)
                n3487 = Multiply(x=1.2 ("y"), y=0.8166) -> (x*y=w4764:dbl)
                n3488 = Multiply(x=1.2 ("y"), y=0.851) -> (x*y=w4769:dbl)
                n3489 = Multiply(x=w4773, y=0.954) -> (x*y=w4780:dbl)
                n3490 = Multiply(x=w4773, y=0.99) -> (x*y=w4783:dbl)
                n3491 = Greater Or Equal?(x=w4784, y=w4783) -> (x >= y?=w4778:bool)
                n3492 = Multiply(x=w4786, y=60.0) -> (x*y=w4792:dbl)
                n3493 = Greater Or Equal?(x=w4784, y=w4780) -> (x >= y?=w4781:bool)
                n3494 = local read "FF 2"() -> (w4787:dbl)
                n3495 = local read item#-1() -> (w4770)
                n3496 = Less?(x=w4770, y=w4764) -> (x < y?=w4767:bool)
                n3497 = In Range and Coerce(upper limit=w4768, x=w4770, lower limit=w4769) -> (In Range?=w4766:bool)  [unwired: 1 out]
                n3498 = Absolute Value(x=w4792) -> (abs(x)=w4790:dbl)
                n3499 = case shown="63.." w4784 {
                  tunnel: [2 3 3 1] -> w4777
                  frame 61, 62 {
                  }
                  frame 63.. {
                  }
                  frame ..0 {
                  }
                  frame 10..60, Default {
                  }
                }
                n3500 = case shown="True" w4778 {
                  tunnel: [1 3] -> w4776
                  frame False {
                  }
                  frame True {
                  }
                }
                n3501 = case shown="True" w4781 {
                  tunnel: [1 2] -> w4775
                  frame False {
                  }
                  frame True {
                  }
                }
                n3502 = Multiply(x=1.2 ("y"), y=0.95) -> (x*y=w4754:dbl)
                n3503 = case shown="1..10, Default" w4788 {
                  tunnel: [1 3] -> w4795
                  frame 1..10, Default {
                  }
                  frame 11.. {
                  }
                }
                n3504 = case shown="0..10, Default" w4787 {
                  tunnel: [1 2 3] -> w4794
                  frame 0..10, Default {
                  }
                  frame 11, 12 {
                  }
                  frame 13.. {
                  }
                }
                n3505 = case shown="3601.." w4790 {
                  tunnel: [1 2 3] -> w4789
                  frame 0..3000, Default {
                    # "Normal"
                  }
                  frame 3001..3600 {
                  }
                  frame 3601.. {
                  }
                }
                n3506 = Or(x=w4767, y=w4766) -> (x .or. y?=w4765:bool)
                n3507 = Greater Or Equal?(x=w4770, y=w4754) -> (x >= y?=w4757:bool)
                n3508 = case shown="0, 1, Default" w4770 {
                  tunnel: [1 3] -> w4753
                  frame 0, 1, Default {
                  }
                  frame 2.. {
                  }
                }
                n3509 = case shown="True" w4757 {
                  tunnel: [1 3] -> w4752
                  frame False {
                  }
                  frame True {
                  }
                }
                n3510 = case shown="True" w4765 {
                  tunnel: [1 2] -> w4751
                  frame False {
                  }
                  frame True {
                  }
                }
                n3511 = Build Array(w4777, w4776, w4775) -> (w4774:i32[])
                n3512 = Number To Decimal String(number=w4789) -> (decimal integer string=→"sp_st":string)  [unwired: 1 in]
                n3513 = Array Max & Min(array=w4774) -> (max value=w4771:i32)  [unwired: 3 out]
                "TEMP STATE" <- w4771
                n3514 = Number To Decimal String(number=w4795) -> (decimal integer string=w4798:string)  [unwired: 1 in]
                n3515 = Number To Decimal String(number=w4794) -> (decimal integer string=w4796:string)  [unwired: 1 in]
                n3516 = Number To Decimal String(number=w4771) -> (decimal integer string=→"temp_st":string)  [unwired: 1 in]
                n3517 = Build Array(w4753, w4752, w4751) -> (w4750:i32[])
                n3518 = local write "nl_st"(w4798) -> ()
                n3519 = local write "ff_st"(w4796) -> ()
                n3520 = Number To Decimal String(number=1) -> (decimal integer string=w4793:string)  [unwired: 1 in]
                n3521 = Array Max & Min(array=w4750) -> (max value=w4749:i32)  [unwired: 3 out]
                n3522 = local write "Air temp"(w4793) -> ()
                n3523 = Number To Decimal String(number=w4749) -> (decimal integer string=w4748:string)  [unwired: 1 in]
                n3524 = local write "Stroke Ln 2"(w4748) -> ()
              }
            }
            n3525 = local read "Stroke Ln 2"() -> (w4660:string)
            n3526 = local read "nl_st"() -> (w4666:string)
            n3527 = local read "ff_st"() -> (w4663:string)
            n3528 = local read "sp_st"() -> (w4664:string)
            n3529 = local read "temp_st"() -> (w4665:string)
            n3530 = local read "Air temp"() -> (w4659:string)
            n3531 = Replace Array Subset(array="in", new element #1=w4666, index #1=1 ("index"), new element #2=w4663, index #2=2 ("index"), new element #3=w4665, index #3=3 ("index"), new element #4=w4664, index #4=4 ("index"), new element #5=w4660, index #5=5 ("index"), new element #6=w4659, index #6=6 ("index"), new element #7="Sensor State" ("new element/subarray"), index #7=0 ("index")) -> (→"out":string[])
          }
        }
        n3532 = Wait (ms)(milliseconds to wait=u32 10) -> ()  [unwired: 1 out]
        n3533 = local read "Quit"() -> (w4654:bool)
      }
      n3534 = while {
        stop <- w4629 stop-if-true
        n3535 = local read "run replace"() -> (w4631:bool)
        n3536 = Wait (ms)(milliseconds to wait=u32 100) -> ()  [unwired: 1 out]
        n3537 = Equal?(x="FLAG 2", y=0.0) -> (x = y?=w4632:bool)
        n3538 = case shown="True" w4632 {
          frame False {
          }
          frame True {
            n3539 = local write "FLAG 2"(100.0 ("FLAG 2")) -> ()
            n3540 = call <vilib>:"Read Characters From File.vi"("file path (dialog if empty)"=path "C:/LAB-IQ-NXT/WO 2449 TT.sig", "convert eol? (no:F)"=FALSE ("append to file? (new file:F)")) -> ("character string"=w4635:string)  [unwired: 4 in, 3 out]
            n3541 = call <vilib>:"Read Characters From File.vi"("file path (dialog if empty)"=path "C:/LAB-IQ-NXT/WO 2449 TRH.sig", "convert eol? (no:F)"=FALSE ("append to file? (new file:F)")) -> ("character string"=w4636:string)  [unwired: 4 in, 3 out]
            n3542 = Decimal String To Number(string=w4635) -> (number=w4637:i32)  [unwired: 2 in, 1 out]
            n3543 = local write "Total No. of Tests"(w4637) -> ()
            n3544 = Decimal String To Number(string=w4636) -> (number=w4640:i32)  [unwired: 2 in, 1 out]
            n3545 = local write "SEN.RUN HRS"(w4640) -> ()
          }
        }
        n3546 = case shown="True" w4631 {
          frame False {
          }
          frame True {
            n3547 = Equal?(x="FLAG 4", y=0.0) -> (x = y?=w4644:bool)
            n3548 = case shown="False" w4644 {
              frame False {
                n3549 = Get Date/Time In Seconds() -> (seconds since 1Jan1904=w4650:timestamp)
                n3550 = local read "START 3"() -> (w4648:dbl)
                n3551 = To Double Precision Float(number=w4650) -> (double precision float=w4649:dbl)
                n3552 = Subtract(x=w4649, y=w4648) -> (x-y=→"SENSOR TIME":dbl)
              }
              frame True {
                n3553 = Get Date/Time In Seconds() -> (seconds since 1Jan1904=w4652:timestamp)
                n3554 = local write "FLAG 4"(100.0 ("FLAG")) -> ()
                n3555 = To Double Precision Float(number=w4652) -> (double precision float=→"START 3":dbl)
              }
            }
          }
        }
        n3556 = local read "Quit"() -> (w4629:bool)
      }
      n3557 = while {
        shift-right: [w4429] -> _
        shift-left: _ -> [w4430]
        tunnel: [w4425] -> _
        i -> [w4425]
        stop <- w4424 stop-if-true
        n3558 = Wait (ms)(milliseconds to wait=u32 50 ("Refresh Rate (ms)")) -> ()  [unwired: 1 out]
        n3559 = local read "Json End Flg"() -> (w4426:bool)
        n3560 = Not(x="Upld AR 2") -> ()  [unwired: 1 out]
        n3561 = local read "Upld AR 2"() -> (w4427:bool)
        n3562 = call "Elapsed Time9"("Time Target (s)"="Sen.Upload Rate (s)", "Reset"=FALSE, "Auto Reset"=TRUE) -> ("Time has Elapsed"=w4436:bool)  [unwired: 9 in, 7 out]
        n3563 = Or(x=w4436, y=w4426) -> (x .or. y?=w4432:bool)
        n3564 = case shown="True" w4432 {
          frame False {
          }
          frame True {
            w4528 = "\"SensorName\":\"" ("string")
            w4498 = " \"},{"
            w4523 = "\",\"SensorState\":\""
            w4525 = "\",\"SensorModelNumber\":\"" ("string")
            w4524 = "\",\"SensorRuntimeHours\":\"" ("string")
            n3565 = local read "model num"() -> (w4522:string[])
            n3566 = local read "Sensor name"() -> (w4541:string[])
            n3567 = local read "run"() -> (w4512:string[])
            n3568 = local read "SENSOR TIME"() -> (w4468:dbl)
            n3569 = local read "out"() -> (w4461:string[])
            n3570 = local read "Total No. of Tests"() -> (w4466:dbl)
            n3571 = Select(t=60.0, s="Run test 3", f=3600.0) -> (s? t:f=w4476:dbl)
            n3572 = Index Array(array=w4522, index #1=1 ("index")) -> (element #1=w4521:string, element #2=w4520:string, element #3=w4519:string, element #4=w4518:string, element #5=w4517:string, element #6=w4516:string)  [unwired: 5 in]
            n3573 = Index Array(array=w4512, index #1=1 ("index")) -> (element #1=w4511:string, element #2=w4510:string, element #3=w4509:string, element #4=w4508:string, element #5=w4507:string, element #6=w4506:string)  [unwired: 5 in]
